vi "Initialize.vi"(8 "error in (no error)":errorcluster, 11 "Console Wrapper in":refnum<class "Console Wrapper.lvclass">) -> (0 "error out":errorcluster, 3 "Console Wrapper out":refnum<class "Console Wrapper.lvclass">)   [LabVIEW 2020, in "Console Wrapper.lvclass"]
doc: "This is a factory method that will encapsulate all complexity needed to start sending the console commands. Initially the required steps you must set the Application Name and the Working directory parameters. If you do not set those values, the Application Name will be empty and the working directory will be C:. It will also pass the command \"dir\" wihtout any options."
uses:
  Console Wrapper.lvclass
  Console Wrapper.lvclass/Console Wrapper.ctl
  Write Application Name.vi
  Write Working Directory.vi
  Write Command.vi
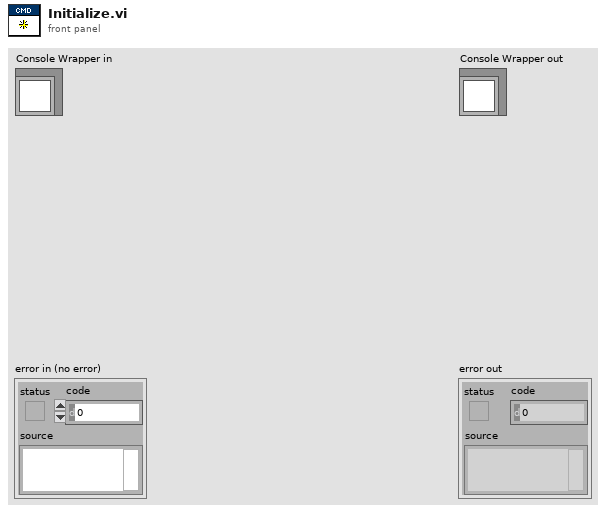
[diagram p1: front panel]
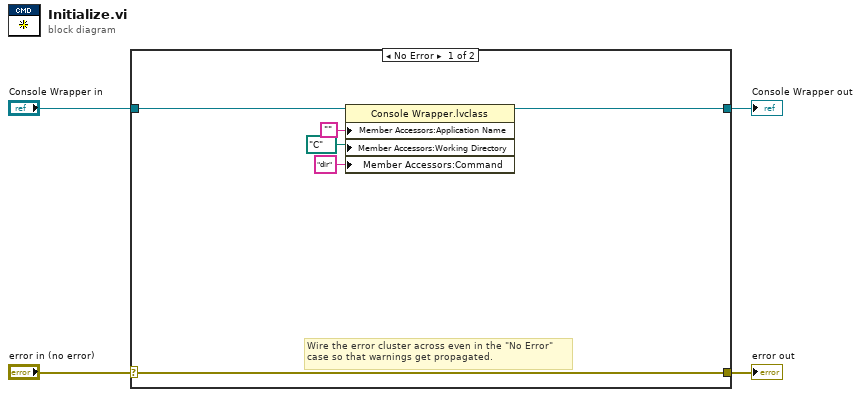
[diagram p0: block diagram]
diagram:
  n1 = case shown="No Error" "error in (no error)" {
    selector: "error in (no error)" -> [w9 w12]
    tunnel: [w9 w12] -> w3
    tunnel: [w8 w11] -> w1
    tunnel: "Console Wrapper in" -> [w10 w11]
    frame No Error {
      # "Wire the error cluster across even in the \"No Error\"\ncase so that warnings get propagated."
      n2 = property class="Console Wrapper.lvclass"(reference=w10, "Member Accessors:Application Name"="", "Member Accessors:Working Directory"=path "C:/" ("Working Directory"), "Member Accessors:Command"="dir" ("Command")) -> (reference out=w8:refnum<class "Console Wrapper.lvclass">)  [unwired: 1 in, 1 out]
    }
    frame Error {
    }
  }
  "error out" <- w3
  "Console Wrapper out" <- w1
